vi "Open.vi"(8 "error in (no error)":errorcluster, 10 "VISA resource name":refnum<visa-resource-name>, 11 "PowerSupply_IT6333A in":refnum<class "PowerSupply_IT6333A.lvclass">) -> (0 "error out":errorcluster, 3 "PowerSupply_IT6333A out":refnum<class "PowerSupply_IT6333A.lvclass">)   [LabVIEW 2017, in "PowerSupply_IT6333A.lvclass"]
uses:
  PowerSupply_IT6333A.lvclass
  <vilib>/Instr/_visa.llb/VISA Open Access Mode.ctl
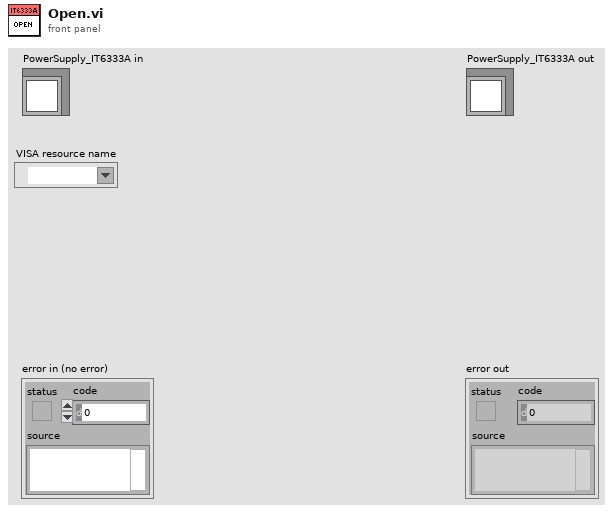
[diagram p1: front panel]
types:
  T1 = typedef "VISA Open Access Mode.ctl" = u32
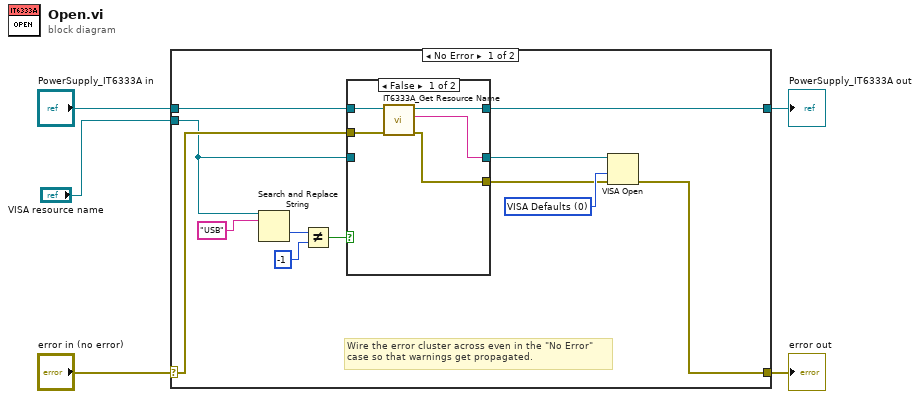
[diagram p0: block diagram]
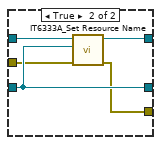
[diagram p2: hidden frame]
diagram:
  n1 = case shown="No Error" "error in (no error)" {
    selector: "error in (no error)" -> [w15 w29]
    tunnel: [w11 w29] -> w4
    tunnel: [w12 w28] -> w2
    tunnel: "PowerSupply_IT6333A in" -> [w16 w28]
    tunnel: "VISA resource name" -> [w10 _]
    frame No Error {
      w17 = T1 0 items=["VISA Defaults"=0, "Exclusive Lock"=1, "Load Configured Settings"=4] ("Access Mode")
      # "Wire the error cluster across even in the \"No Error\"\ncase so that warnings get propagated."
      n2 = Search and Replace String(input string=w10, search string="USB") -> (offset past replacement=w7:i32)  [unwired: 6 in, 3 out]
      n3 = Not Equal?(x=w7, y=-1) -> (x != y?=w9:bool)
      n4 = case shown="False" w9 {
        tunnel: w16 -> [w22 w27]
        tunnel: w15 -> [w21 w24]
        tunnel: [w20 w23] -> w14
        tunnel: [w19 w25] -> w13
        tunnel: [w18 w26] -> w12
        tunnel: w10 -> [_ w25]
        frame False {
          n5 = call-dynamic "IT6333A_Get Resource Name.vi"("error in (no error)"=w21, "PowerSupply_IT6333A in"=w22) -> ("error out"=w20:errorcluster, "Resource Name"=w19:string, "PowerSupply_IT6333A out"=w18:refnum<class "PowerSupply_IT6333A.lvclass">)  [unwired: 7 in]
        }
        frame True {
          n6 = call-dynamic "IT6333A_Set Resource Name.vi"("error in (no error)"=w24, "Resource Name"=w25, "PowerSupply_IT6333A in"=w27) -> ("error out"=w23:errorcluster, "PowerSupply_IT6333A out"=w26:refnum<class "PowerSupply_IT6333A.lvclass">)  [unwired: 7 in]
        }
      }
      n7 = VISA Open(access mode=w17, error in (no error)=w14, VISA resource name=w13) -> (error out=w11:errorcluster)  [unwired: 2 in, 1 out]
    }
    frame Error {
    }
  }
  "error out" <- w4
  "PowerSupply_IT6333A out" <- w2
